vi "Duplicate Cut 2012 NIVerified.vi"(11 "Array In":string[](array[string])) -> (3 "Array Out":string[](array[string]))   [LabVIEW 2018]
panel:
  # "Overview\nRemoves duplicate strings in a 1 dimensional string array and returns the reduced array unsorted.\nRequirements\nLabVIEW 2012( or compatible)\nInstructions\n1.\tDownload the VI\n2.\tWire a string array to the Array In terminal\n3.\tRun the VI and take the reduced array from the Array Out terminal."
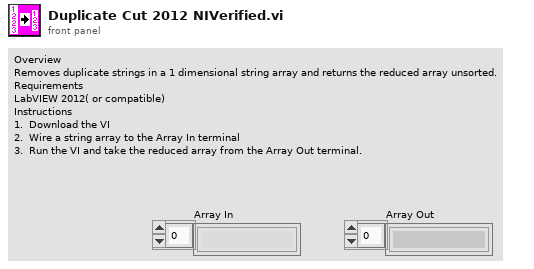
[diagram p1: front panel]
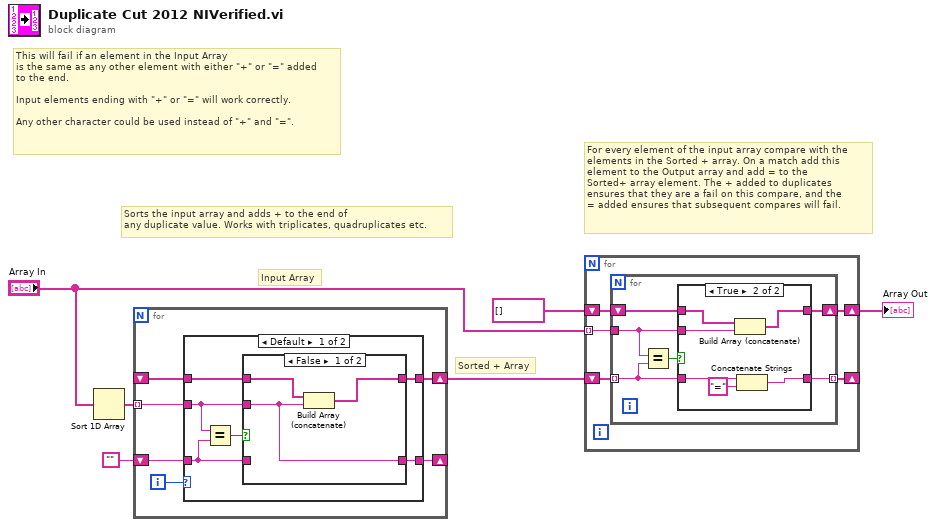
[diagram p0: block diagram]
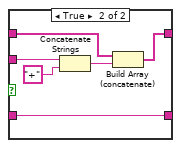
[diagram p3: hidden frame]
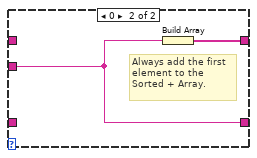
[diagram p4: hidden frame]
diagram:
  # "Input Array"
  # "This will fail if an element in the Input Array\nis the same as any other element with either \"+\" or \"=\" added\nto the end.\n\nInput elements ending with \"+\" or \"=\" will work correctly.\n\nAny other character could be used instead of \"+\" and \"=\"."
  # "For every element of the input array compare with the\nelements in the Sorted + array. On a match add this\nelement to the Output array and add = to the\nSorted+ array element. The + added to duplicates\nensures that they are a fail on this compare, and the \n= added ensures that subsequent compares will fail."
  # "Sorted + Array"
  # "Sorts the input array and adds + to the end of\nany duplicate value. Works with triplicates, quadruplicates etc."
  n1 = Sort 1D Array(array="Array In") -> (sorted array=w5:string[])
  n2 = for {
    tunnel: w5 -> [w12] mode=indexing
    shift-right: [w10] -> _
    shift-left: "" -> [w9]
    shift-right: [w11] -> w4
    shift-left: _ -> [w8]
    i -> [w7]
    n3 = case shown="Default" w7 {
      tunnel: w12 -> [w15 w28]
      tunnel: [w16 w29] -> w11
      tunnel: [w18 w28] -> w10
      tunnel: w9 -> [w14 _]
      tunnel: w8 -> [w17 _]
      frame Default {
        n4 = Equal?(x=w15, y=w14) -> (x = y?=w13:bool)
        n5 = case shown="False" w13 {
          tunnel: w14 -> [_ w27]
          tunnel: [w19 w27] -> w18
          tunnel: [w20 w22] -> w16
          tunnel: w17 -> [w21 w23]
          tunnel: w15 -> [w19 w26]
          frame False {
            n6 = Build Array (concatenate)(w21, w19) -> (w20:string[])
          }
          frame True {
            n7 = Concatenate Strings(w26, "+") -> (w24:string)
            n8 = Build Array (concatenate)(w23, w24) -> (w22:string[])
          }
        }
      }
      frame 0 {
        # "Always add the first\nelement to the\nSorted + Array."
        n9 = Build Array(w28) -> (w29:string[])
      }
    }
  }
  n10 = for {
    tunnel: "Array In" -> [w34] mode=indexing
    shift-right: [w31] -> w1
    shift-left: string[] [] ("appended array") -> [w32]
    shift-right: [w30] -> _
    shift-left: w4 -> [w33]
    n11 = for {
      tunnel: w34 -> [w35]
      tunnel: w33 -> [w36] mode=indexing
      tunnel: [w37] -> w30 mode=indexing
      shift-right: [w38] -> w31
      shift-left: w32 -> [w40]
      n12 = Equal?(x=w35, y=w36) -> (x = y?=w39:bool)
      n13 = case shown="True" w39 {
        tunnel: w40 -> [w42 w48]
        tunnel: w35 -> [_ w47]
        tunnel: [w42 w46] -> w38
        tunnel: w36 -> [w41 w44]
        tunnel: [w41 w43] -> w37
        frame False {
        }
        frame True {
          n14 = Build Array (concatenate)(w48, w47) -> (w46:string[])
          n15 = Concatenate Strings(w44, "=" ("string")) -> (w43:string)
        }
      }
    }
  }
  "Array Out" <- w1
